vi "PITerminal.vi"(0 "System no.":i32=1 min=1 max=4 step=1, 1 "String to Send":string) -> (14 "Comm Window":string)   [LabVIEW 2020]
doc: "Simple Terminal Application.\nThis VI can be executed in parallel to any existing PI LabVIEW application. \nIf not already connected to a PI device, PI_GCS2_Configuration_Setup.vi is opened automatically. Please use PI_GCS2_Configuration_Setup.vi to connect to your PI GCS2 device.\n\nShortcut keys:\nReturn: Send or query\nF5: ERR? (with error translation)\nF12: Additional receive function (e.g. to clear output buffer of the connected device)\nPage Up: Command history previous entry\nPage down: Command history next entry"
uses:
  Low Level/Communication.llb/Global1.vi
panel:
  in  "F5":bool
  in  "Command History":string[](array[string])
  in  "Receive":bool
  out "History length":i32
  in  "History DOWN":bool
  in  "History Index":i32
  in  "History UP":bool
  in  "Send":bool
  in  "Clear":bool
  in  "stop":bool
  # "PITerminal"
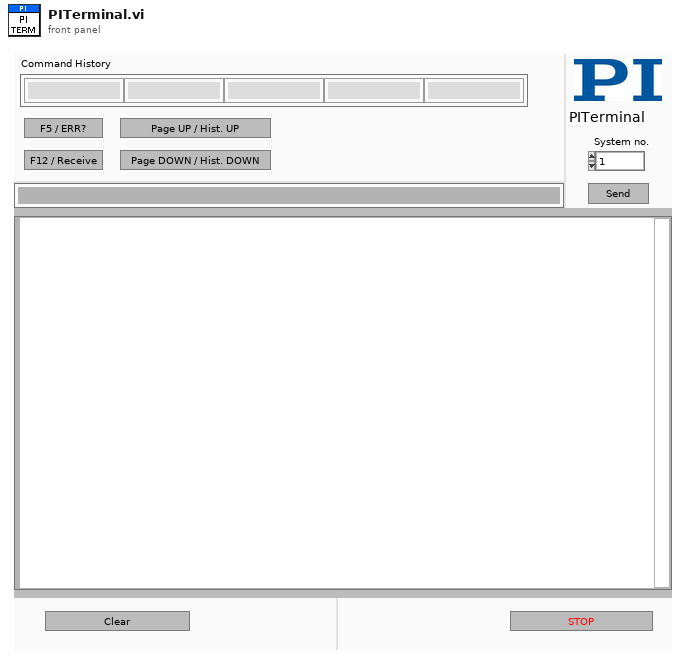
[diagram p1: front panel]
types:
  T1 = enum32{"Invalid", "Standard", "Closed", "Hidden", "Minimized", "Maximized"}
  T2 = enum16{"Disable error check", "Force error check", "Use global settings"}
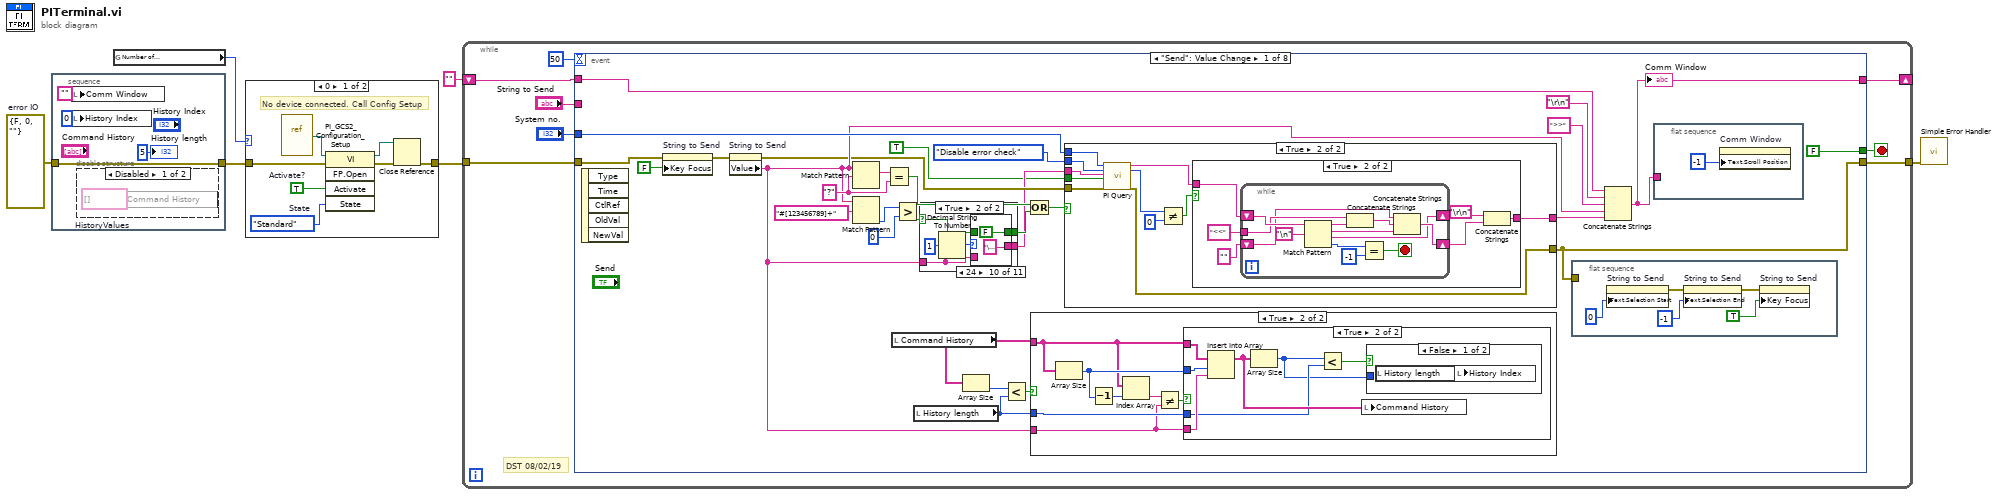
[diagram p0: block diagram]
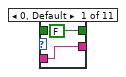
[diagram p5: hidden frame]
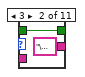
[diagram p6: hidden frame]
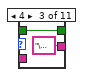
[diagram p7: hidden frame]
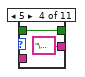
[diagram p8: hidden frame]
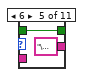
[diagram p9: hidden frame]
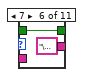
[diagram p10: hidden frame]
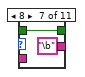
[diagram p11: hidden frame]
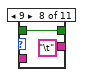
[diagram p12: hidden frame]
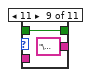
[diagram p13: hidden frame]
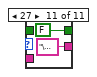
[diagram p14: hidden frame]
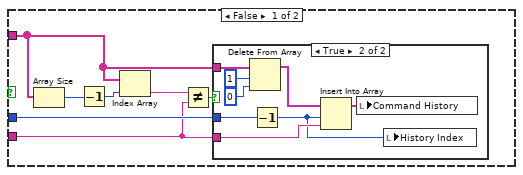
[diagram p15: hidden frame]
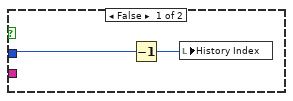
[diagram p16: hidden frame]
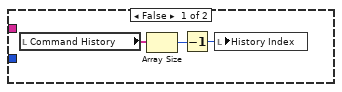
[diagram p17: hidden frame]
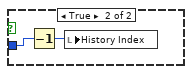
[diagram p18: hidden frame]
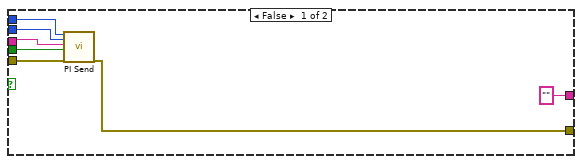
[diagram p19: hidden frame]
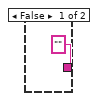
[diagram p20: hidden frame]
diagram:
  w4 = errorcluster {"status"=FALSE, "code"=0, "source"=""}  # error IO
  n1 = stacked-sequence {
    tunnel: w4 -> [w9]
    tunnel: [w9] -> w3
    frame #0 {
      n2 = local write "History Index"(0) -> ()
      n3 = local write "Comm Window"("") -> ()
      n4 = disable-structure shown="Disabled" {
        frame Disabled {
          w11 = string[] []  # HistoryValues
          n5 = local write "Command History"(w11) -> ()
        }
        frame Enabled {
        }
      }
      "History length" <- 5
    }
  }
  n6 = global read "Global1.vi" "Number of\nsystems"() -> (w1:i32)
  n7 = case shown="0" w1 {
    tunnel: w3 -> [w16 w19]
    tunnel: [w14 w19] -> w2
    frame 0 {
      w17 = T1."Standard"  # State
      w15 = TRUE  # Activate?
      # "No device connected. Call Config Setup"
      n8 = vi-ref "PI_GCS2_Configuration_Setup.vi"() -> (w18:refnum<vi>)
      n9 = invoke class="VI" method="FP.Open"(reference=w18, error in=w16, "Activate"=w15, "State"=w17) -> (reference out=w12:refnum<vi>, error out=w13:errorcluster)  [unwired: 1 in, 3 out]
      n10 = Close Reference(reference=w12, error in (no error)=w13) -> (error out=w14:errorcluster)
    }
    frame 1, Default {
      # "At least 1 device connected.\nNothing to do here..."
    }
  }
  n11 = while {
    tunnel: [w26] -> w6
    tunnel: w2 -> [w24]
    shift-right: [w23] -> _
    shift-left: "" -> [w20]
    stop <- w22 stop-if-true
    # "DST 08/02/19"
    n12 = event shown="[0] \"Send\": Value Change" {
      selector: _ -> [_ _ _ _ _ _ _ _]
      dyn-events: _ -> [_ _ _ _ _ _ _ _]
      timeout: 50 -> [_ _ _ _ _ _ _ _]
      tunnel: "String to Send" -> [_ _ _ _ _ _ _ _]
      tunnel: [w46 w169 w216 w238 w247 w269 w276 w279] -> w23
      tunnel: [w33 w167 w211 w232 w242 w265 w275 w278] -> w26
      tunnel: "System no." -> [w56 w171 w213 _ _ _ _ _]
      tunnel: w24 -> [w45 w172 w214 w231 w242 w265 w275 w278]
      tunnel: [FALSE FALSE FALSE FALSE FALSE FALSE FALSE "stop"] -> w22
      tunnel: w20 -> [w55 w170 w215 _ w247 w269 w276 w279]
      event "Send": Value Change {
        w49 = "?"
        n13 = event-data() -> ()  [unwired: 6 out]
        n14 = property on="String to Send" class="Str"(error in=w45, "Key Focus"=FALSE) -> (error out=w43:errorcluster)  [unwired: 1 in, 1 out]
        n15 = property on="String to Send" class="Str"(error in=w43) -> (error out=w31:errorcluster, "Value"=w36:string)  [unwired: 1 in, 1 out]
        n16 = Match Pattern(string=w36, regular expression=w49) -> (match substring=w51:string)  [unwired: 4 out]
        n17 = Match Pattern(string=w36, regular expression="#[123456789]+") -> (offset past match=w38:i32)  [unwired: 4 out]
        n18 = Equal?(x=w51, y=w49) -> (x = y?=w48:bool)
        n19 = local read "Command History"() -> (w40:string[])
        n20 = Greater?(x=w38, y=0) -> (0:w35:bool)
        n21 = local read "History length"() -> (w39:i32)
        n22 = case shown="True" w35 {
          selector: w35 -> [w62 w65]
          tunnel: w36 -> [w63 w66]
          tunnel: [w63 w67] -> w30
          tunnel: [w62 w64] -> w32
          frame False {
          }
          frame True {
            n23 = Decimal String To Number(string=w66, offset=1) -> (number=w68:i32)  [unwired: 2 out]
            n24 = case shown="24" w68 {
              tunnel: [w71 "\u0003" "\u0004" "\u0005" "\u0006" "\u0007" "\b" "\t" "\u000b" "\u0018" "\u001b"] -> w67
              tunnel: w66 -> [w71 _ _ _ _ _ _ _ _ _ _]
              tunnel: w65 -> [_ w72 w74 w76 w78 w80 w82 w84 w86 _ _]
              tunnel: [FALSE w72 w74 w76 w78 w80 w82 w84 w86 FALSE FALSE] -> w64
              frame 0, Default {
              }
              frame 3 {
              }
              frame 4 {
              }
              frame 5 {
              }
              frame 6 {
              }
              frame 7 {
              }
              frame 8 {
              }
              frame 9 {
              }
              frame 11 {
              }
              frame 24 {
              }
              frame 27 {
              }
            }
          }
        }
        n25 = Array Size(array=w40) -> (size(s)=w42:i32)
        n26 = Less?(x=w42, y=w39) -> (x < y?=w41:bool)
        n27 = Or(x=w48, y=w32) -> (x .or. y?=w47:bool)
        n28 = case shown="True" w41 {
          tunnel: w36 -> [w93 w110]
          tunnel: w40 -> [w97 w112]
          tunnel: w39 -> [w98 w115]
          frame False {
            n29 = Array Size(array=w97) -> (size(s)=w95:i32)
            n30 = Decrement(x=w95) -> (x-1=w96:i32)
            n31 = Index Array(array=w97, index=w96) -> (element=w94:string)
            n32 = Not Equal?(x=w94, y=w93) -> (x != y?=w92:bool)
            n33 = case shown="True" w92 {
              tunnel: w97 -> [_ w108]
              tunnel: w93 -> [_ w105]
              tunnel: w98 -> [w100 w102]
              frame False {
                n34 = Decrement(x=w100) -> (x-1=w99:i32)
                n35 = local write "History Index"(w99) -> ()
              }
              frame True {
                n36 = Delete From Array(array=w108, length=1, index=0) -> (array with subset deleted=w106:string[])  [unwired: 1 out]
                n37 = Decrement(x=w102) -> (x-1=w101:i32)
                n38 = Insert Into Array(array=w106, index=w101, new element=w105) -> (w104:string[])
                n39 = local write "Command History"(w104) -> ()
                n40 = local write "History Index"(w101) -> ()
              }
            }
          }
          frame True {
            n41 = Array Size(array=w112) -> (size(s)=w114:i32)
            n42 = Decrement(x=w114) -> (x-1=w113:i32)
            n43 = Index Array(array=w112, index=w113) -> (element=w111:string)
            n44 = Not Equal?(x=w111, y=w110) -> (x != y?=w109:bool)
            n45 = case shown="True" w109 {
              tunnel: w112 -> [_ w125]
              tunnel: w110 -> [_ w124]
              tunnel: w114 -> [_ w123]
              tunnel: w115 -> [_ w121]
              frame False {
                n46 = local read "Command History"() -> (w118:string[])
                n47 = Array Size(array=w118) -> (size(s)=w117:i32)
                n48 = Decrement(x=w117) -> (x-1=w116:i32)
                n49 = local write "History Index"(w116) -> ()
              }
              frame True {
                n50 = Insert Into Array(array=w125, index=w123, new element=w124) -> (w122:string[])
                n51 = Array Size(array=w122) -> (size(s)=w119:i32)
                n52 = Less?(x=w119, y=w121) -> (x < y?=w120:bool)
                n53 = local write "Command History"(w122) -> ()
                n54 = case shown="False" w120 {
                  tunnel: w119 -> [_ w127]
                  frame False {
                    n55 = local read "History length"() -> (w126:i32)
                    n56 = local write "History Index"(w126) -> ()
                  }
                  frame True {
                    n57 = Decrement(x=w127) -> (x-1=w128:i32)
                    n58 = local write "History Index"(w128) -> ()
                  }
                }
              }
            }
          }
        }
        n59 = case shown="True" w47 {
          tunnel: w31 -> [w134 w141]
          tunnel: [w133 w140] -> w33
          tunnel: w56 -> [w135 w144]
          tunnel: ["" w145] -> w52
          tunnel: w30 -> [w132 w139]
          tunnel: TRUE ("Attach Linefeed?") -> [w131 w138]
          tunnel: T2."Disable error check" ("Error check settings") -> [w130 w137]
          frame False {
            n60 = call "PI Send.vi"("System no."=w135, "Error check settings"=w130, "String to send"=w132, "Attach termination char.?"=w131, "error in"=w134) -> ("error out"=w133:errorcluster)  [unwired: 1 in, 13 out]
          }
          frame True {
            n61 = call "PI Query.vi"("System no."=w144, "Error check settings"=w137, "String to send"=w139, "Attach termination char.?"=w138, "error in"=w141) -> ("String read"=w143:string, "bytes read"=w142:u16, "error out"=w140:errorcluster)  [unwired: 2 in, 10 out]
            n62 = Not Equal?(x=w142, y=u16 0) -> (x != y?=w147:bool)
            n63 = case shown="True" w147 {
              tunnel: w143 -> [_ w154]
              tunnel: ["" w149] -> w145
              frame False {
              }
              frame True {
                n64 = while {
                  tunnel: "<<" -> [w161]
                  shift-right: [w159] -> w150
                  shift-left: "" -> [w157]
                  shift-right: [w158] -> _
                  shift-left: w154 -> [w166]
                  stop <- w162 stop-if-true
                  n65 = Match Pattern(string=w166, regular expression="\n") -> (before substring=w160:string, match substring=w155:string, after substring=w158:string, offset past match=w164:i32)  [unwired: 1 out]
                  n66 = Concatenate Strings(w161, w160) -> (w156:string)
                  n67 = Equal?(x=w164, y=-1) -> (x = y?=w162:bool)
                  n68 = Concatenate Strings(w157, w156, w155) -> (w159:string)
                }
                n69 = Concatenate Strings("\r\n", w150) -> (w149:string)
              }
            }
          }
        }
        n70 = flat-sequence {
          tunnel: w33 -> [_]
          frame #0 {
            n71 = property on="String to Send" class="Str"("Text.Selection Start"=u32 0 ("Text.Selection:Start")) -> (error out=w59:errorcluster)  [unwired: 2 in, 1 out]
            n72 = property on="String to Send" class="Str"(error in=w59, "Text.Selection End"=-1) -> (error out=w58:errorcluster)  [unwired: 1 in, 1 out]
            n73 = property on="String to Send" class="Str"(error in=w58, "Key Focus"=TRUE) -> ()  [unwired: 1 in, 2 out]
          }
        }
        n74 = Concatenate Strings(w55, "\r\n", ">>", w36, w52) -> (w46:string)
        "Comm Window" <- w46
        n75 = flat-sequence {
          tunnel: w46 -> [_]
          frame #0 {
            n76 = property on="Comm Window" class="Str"("Text.Scroll Position"=-1) -> ()  [unwired: 2 in, 2 out]
          }
        }
      }
      event "Receive": Value Change {
        n77 = event-data() -> ()  [unwired: 7 out]
        n78 = call "PI Receive String.vi"("System no."=w171, "error in"=w172) -> ("String read"=w176:string, "bytes read"=w175:u16, "error out"=w167:errorcluster)  [unwired: 1 in, 14 out]
        n79 = Not Equal?(x=w175, y=u16 0) -> (x != y?=w174:bool)
        n80 = case shown="True" w174 {
          tunnel: w176 -> [_ w189]
          tunnel: ["" w184] -> w177
          frame False {
          }
          frame True {
            n81 = while {
              tunnel: "<<" -> [w196]
              shift-right: [w194] -> w185
              shift-left: "" -> [w192]
              shift-right: [w193] -> _
              shift-left: w189 -> [w201]
              stop <- w197 stop-if-true
              n82 = Match Pattern(string=w201, regular expression="\n") -> (before substring=w195:string, match substring=w190:string, after substring=w193:string, offset past match=w199:i32)  [unwired: 1 out]
              n83 = Concatenate Strings(w196, w195) -> (w191:string)
              n84 = Equal?(x=w199, y=-1) -> (x = y?=w197:bool)
              n85 = Concatenate Strings(w192, w191, w190) -> (w194:string)
            }
            n86 = Concatenate Strings("\r\n", w185) -> (w184:string)
          }
        }
        n87 = Concatenate Strings(w170, w177) -> (w169:string)
        n88 = flat-sequence {
          tunnel: w167 -> [_]
          frame #0 {
            w181 = u32 0  # Text.Selection:Start
            n89 = property on="String to Send" class="Str"("Text.Selection Start"=w181) -> (error out=w180:errorcluster)  [unwired: 2 in, 1 out]
            n90 = property on="String to Send" class="Str"(error in=w180, "Text.Selection End"=-1) -> (error out=w179:errorcluster)  [unwired: 1 in, 1 out]
            n91 = property on="String to Send" class="Str"(error in=w179, "Key Focus"=TRUE) -> ()  [unwired: 1 in, 2 out]
          }
        }
        n92 = local write "Comm Window"(w169) -> ()
        n93 = flat-sequence {
          tunnel: w169 -> [_]
          frame #0 {
            n94 = property on="Comm Window" class="Str"("Text.Scroll Position"=-1) -> ()  [unwired: 2 in, 2 out]
          }
        }
      }
      event "F5": Value Change {
        n95 = event-data() -> ()  [unwired: 7 out]
        n96 = call "ERR_Query.vi"("System no."=w213, "error in"=w214) -> ("error out"=w206:errorcluster)  [unwired: 17 out]
        n97 = call "GCSTranslateError.vi"("error in"=w206) -> ("Error Description"=w207:string, "error out"=w212:errorcluster)  [unwired: 17 out]
        n98 = Unbundle By Name(w206) -> ("code"=w204:i32)
        n99 = Equal?(x=w204, y=0) -> (x = y?=w209:bool)
        n100 = case shown="False" w209 {
          tunnel: w207 -> [w221 _]
          tunnel: [w226 "<<0  -  (error 0 - \"No error\")"] -> w208
          tunnel: w204 -> [w225 _]
          frame False {
            n101 = Number To Decimal String(number=w225) -> (decimal integer string=w223:string)  [unwired: 1 out]
            n102 = Concatenate Strings("<<", w223, "  -  (error ", w223, " - \"", w221, "\")") -> (w226:string)
          }
          frame True {
          }
        }
        n103 = Concatenate Strings(w215, "\r\n", ">>", "ERR?", "\r\n", w208) -> (w216:string)
        n104 = flat-sequence {
          tunnel: w216 -> [_]
          frame #0 {
            n105 = property on="Comm Window" class="Str"("Text.Scroll Position"=-1) -> ()  [unwired: 2 in, 2 out]
          }
        }
        n106 = local write "Comm Window"(w216) -> ()
        n107 = call <vilib>:"Clear Errors.vi"("error in (no error)"=w212) -> ("error out"=w211:errorcluster)  [unwired: 1 in, 5 out]
      }
      event "Clear": Value Change {
        w236 = u32 0  # Text.Selection:Start
        w238 = ""
        n108 = event-data() -> ()  [unwired: 7 out]
        n109 = property on="String to Send" class="Str"(error in=w231, "Text.Selection Start"=w236) -> (error out=w234:errorcluster)  [unwired: 1 in, 1 out]
        n110 = property on="String to Send" class="Str"(error in=w234, "Text.Selection End"=-1) -> (error out=w233:errorcluster)  [unwired: 1 in, 1 out]
        n111 = property on="String to Send" class="Str"(error in=w233, "Key Focus"=TRUE) -> (error out=w232:errorcluster)  [unwired: 1 in, 1 out]
        n112 = local write "Comm Window"(w238) -> ()
      }
      event "History UP": Value Change {
        n113 = event-data() -> ()  [unwired: 7 out]
        n114 = local read "History Index"() -> (w246:i32)
        n115 = local read "Command History"() -> (w241:string[])
        n116 = Less?(x=w246, y=1) -> (x < y?=w244:bool)
        n117 = case shown="False" w244 {
          tunnel: [w253 0] -> w240
          tunnel: w246 -> [w251 _]
          tunnel: w241 -> [w252 _]
          frame False {
            n118 = Index Array(array=w252, index=w251) -> (element=w250:string)
            n119 = Not Equal?(x=w250, y="") -> (x != y?=w248:bool)
            n120 = case shown="False" w248 {
              tunnel: [w254 w258] -> w253
              tunnel: w251 -> [w256 w257]
              frame False {
                n121 = Decrement(x=w256) -> (x-1=w255:i32)
                n122 = Decrement(x=w255) -> (x-1=w254:i32)
              }
              frame True {
                n123 = Decrement(x=w257) -> (x-1=w258:i32)
              }
            }
          }
          frame True {
          }
        }
        n124 = Index Array(array=w241, index=w240) -> (element=w243:string)
        n125 = local write "History Index"(w240) -> ()
        n126 = local write "String to Send"(w243) -> ()
      }
      event "History DOWN": Value Change {
        n127 = event-data() -> ()  [unwired: 7 out]
        n128 = local read "Command History"() -> (w264:string[])
        n129 = Array Size(array=w264) -> (size(s)=w263:i32)
        n130 = Decrement(x=w263) -> (x-1=w261:i32)
        n131 = local read "History Index"() -> (w268:i32)
        n132 = Decrement(x=w261) -> (x-1=w262:i32)
        n133 = Greater?(x=w268, y=w262) -> (0:w267:bool)
        n134 = case shown="True" w267 {
          tunnel: [w272 w273] -> w270
          tunnel: w268 -> [w271 _]
          tunnel: w261 -> [_ w273]
          frame False {
            n135 = Increment(x=w271) -> (x+1=w272:i32)
          }
          frame True {
          }
        }
        n136 = local write "History Index"(w270) -> ()
        n137 = Index Array(array=w264, index=w270) -> (element=w266:string)
        n138 = local write "String to Send"(w266) -> ()
      }
      event Timeout {
        n139 = event-data() -> ()  [unwired: 4 out]
      }
      event "stop": Value Change {
        n140 = event-data() -> ()  [unwired: 4 out]
      }
    }
  }
  n141 = call <vilib>:"Simple Error Handler.vi"("error in (no error)"=w6) -> ()  [unwired: 1 in, 8 out]
